vi "FT10_Semi-Auto Deactivate Port.vi"(7 "Wait Time (ms)":i32=10, 9 "Mode in":T2, 10 "Port in":T1) -> (1 "Mode out":T2, 2 "Port out":T1, 3 "Command Cluster":T3)   [LabVIEW 2015]
doc: "Creates message for Message Handling Loop to deactivate specified port."
uses:
  Controls/Control_Command Cluster.ctl
  Controls/Control_Semi-Auto Port.ctl
  Controls/Control_Semi-Auto Mode.ctl
  Controls/Control_Fornax Mono1 Cut Activate Port Bool.ctl
  Controls/Control_Fornax Mono1 Coag Activate Port Bool.ctl
  Controls/Control_Fornax Mono2 Cut Activate Port Bool.ctl
  Controls/Control_Fornax Mono2 Coag Activate Port Bool.ctl
  Controls/Control_Fornax Bipolar Activate Port Bool.ctl
  Controls/Control_Fornax Ligasure Activate Port Bool.ctl
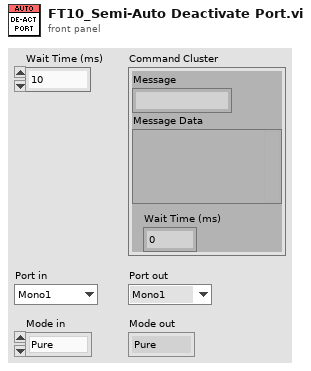
[diagram p1: front panel]
types:
  T1 = typedef "Control_Semi-Auto Port.ctl" = enum16{"Mono1", "Mono2", "Bipolar", "Ligasure", "Error"}
  T2 = typedef "Control_Semi-Auto Mode.ctl" = enum16{"Pure", "Blend", "Spray", "Fulgerate", "Standard", "Macro", "Precision", "Ligasure", "Error"}
  T3 = typedef "Control_Command Cluster.ctl" = cluster{"Message":string, "Message Data":variant, "Wait Time (ms)":i32}
  T4 = typedef "Control_Fornax Mono1 Coag Activate Port Bool.ctl" = bool
  T5 = typedef "Control_Fornax Mono2 Coag Activate Port Bool.ctl" = bool
  T6 = typedef "Control_Fornax Mono1 Cut Activate Port Bool.ctl" = bool
  T7 = typedef "Control_Fornax Mono2 Cut Activate Port Bool.ctl" = bool
  T8 = typedef "Control_Fornax Bipolar Activate Port Bool.ctl" = bool
  T9 = typedef "Control_Fornax Ligasure Activate Port Bool.ctl" = bool
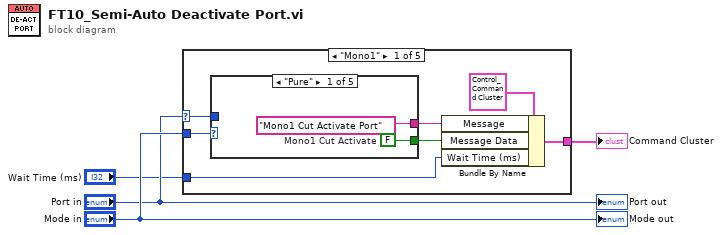
[diagram p0: block diagram]
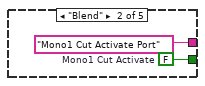
[diagram p2: hidden frame]
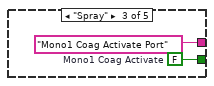
[diagram p3: hidden frame]
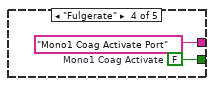
[diagram p4: hidden frame]
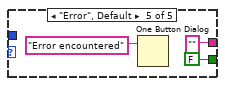
[diagram p5: hidden frame]
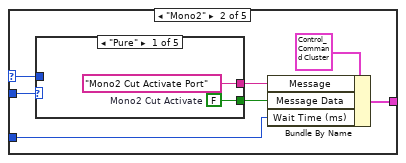
[diagram p6: hidden frame]
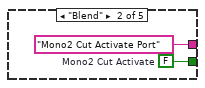
[diagram p7: hidden frame]
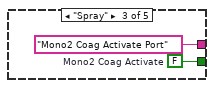
[diagram p8: hidden frame]
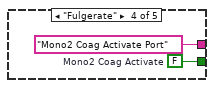
[diagram p9: hidden frame]
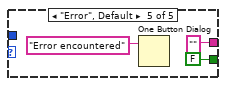
[diagram p10: hidden frame]
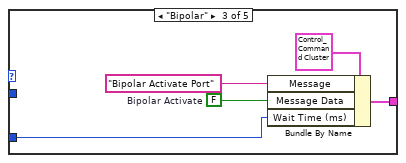
[diagram p11: hidden frame]
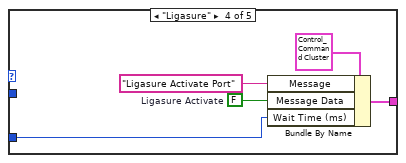
[diagram p12: hidden frame]
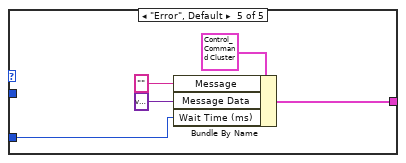
[diagram p13: hidden frame]
diagram:
  n1 = case shown="\"Mono1\"" "Port in" {
    selector: "Port in" -> [w8 w26 _ _ _]
    tunnel: "Mode in" -> [w7 w25 _ _ _]
    tunnel: [w9 w27 w43 w48 w52] -> w2
    tunnel: "Wait Time (ms)" -> [w5 w23 w41 w46 w51]
    frame "Mono1" {
      n2 = case shown="\"Pure\"" w7 {
        tunnel: w8 -> [_ _ _ _ _]
        tunnel: ["Mono1 Cut Activate Port" ("Message") "Mono1 Cut Activate Port" ("Message") "Mono1 Coag Activate Port" ("Message") "Mono1 Coag Activate Port" ("Message") "" ("Message")] -> w10
        tunnel: [w12 w14 w16 w18 T4 FALSE ("Mono1 Coag Activate")] -> w6
        frame "Pure" {
          w12 = T6 FALSE  # Mono1 Cut Activate
        }
        frame "Blend" {
          w14 = T6 FALSE  # Mono1 Cut Activate
        }
        frame "Spray" {
          w16 = T4 FALSE  # Mono1 Coag Activate
        }
        frame "Fulgerate" {
          w18 = T4 FALSE  # Mono1 Coag Activate
        }
        frame "Error", Default {
          n3 = One Button Dialog(message="Error encountered") -> ()  [unwired: 1 in, 1 out]
        }
      }
      n4 = Bundle By Name(cluster=T3 {"Message"="", "Message Data"=variant, "Wait Time (ms)"=0}, "Message"=w10, "Message Data"=w6, "Wait Time (ms)"=w5) -> (w9:T3)
    }
    frame "Mono2" {
      n5 = case shown="\"Pure\"" w25 {
        tunnel: w26 -> [_ _ _ _ _]
        tunnel: ["Mono2 Cut Activate Port" ("Message") "Mono2 Cut Activate Port" ("Message") "Mono2 Coag Activate Port" ("Message") "Mono2 Coag Activate Port" ("Message") "" ("Message")] -> w28
        tunnel: [w30 w32 w34 w36 T5 FALSE ("Mono2 Coag Activate")] -> w24
        frame "Pure" {
          w30 = T7 FALSE  # Mono2 Cut Activate
        }
        frame "Blend" {
          w32 = T7 FALSE  # Mono2 Cut Activate
        }
        frame "Spray" {
          w34 = T5 FALSE  # Mono2 Coag Activate
        }
        frame "Fulgerate" {
          w36 = T5 FALSE  # Mono2 Coag Activate
        }
        frame "Error", Default {
          n6 = One Button Dialog(message="Error encountered") -> ()  [unwired: 1 in, 1 out]
        }
      }
      n7 = Bundle By Name(cluster=T3 {"Message"="", "Message Data"=variant, "Wait Time (ms)"=0}, "Message"=w28, "Message Data"=w24, "Wait Time (ms)"=w23) -> (w27:T3)
    }
    frame "Bipolar" {
      w42 = T8 FALSE  # Bipolar Activate
      n8 = Bundle By Name(cluster=T3 {"Message"="", "Message Data"=variant, "Wait Time (ms)"=0}, "Message"="Bipolar Activate Port", "Message Data"=w42, "Wait Time (ms)"=w41) -> (w43:T3)
    }
    frame "Ligasure" {
      w47 = T9 FALSE  # Ligasure Activate
      n9 = Bundle By Name(cluster=T3 {"Message"="", "Message Data"=variant, "Wait Time (ms)"=0}, "Message"="Ligasure Activate Port", "Message Data"=w47, "Wait Time (ms)"=w46) -> (w48:T3)
    }
    frame "Error", Default {
      n10 = Bundle By Name(cluster=T3 {"Message"="", "Message Data"=variant, "Wait Time (ms)"=0}, "Message"="", "Message Data"=variant, "Wait Time (ms)"=w51) -> (w52:T3)
    }
  }
  "Command Cluster" <- w2
  "Port out" <- "Port in"
  "Mode out" <- "Mode in"
